vi "VoltageBlocks.vi"() -> ()   [LabVIEW 2011]
uses:
  <vilib>/DAQmx/write.llb/DAQmx Write (Analog 1D DBL NChan 1Samp).vi
  <vilib>/DAQmx/create/channels.llb/DAQmx Create Channel (AO-Voltage-Basic).vi
  <vilib>/DAQmx/miscellaneous.llb/DAQmx Fill In Error Info.vi
panel:
  in  "data":dbl[](array[slide]) scale=0.0..4.5
  in  "physical channels":tag
  out "Waveform Chart":dynamicdata(graph)
  in  "stop":bool
  in  "maximum value":dbl=5.0 format="%0.2f"
  in  "minimum value":dbl=-5.0 format="%0.2f"
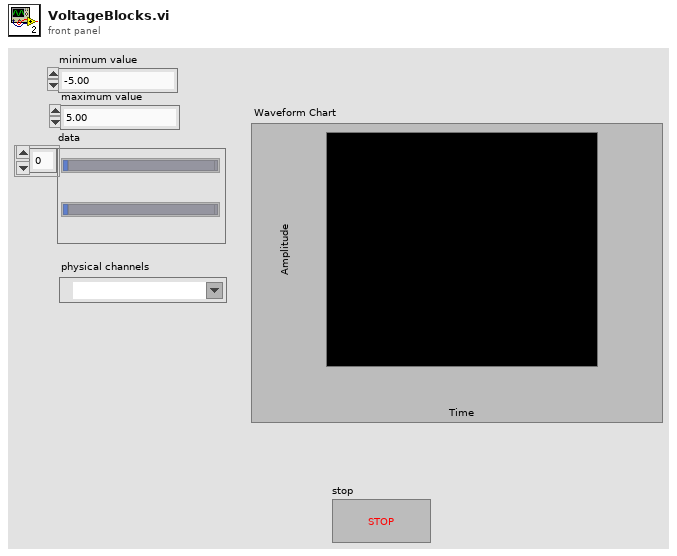
[diagram p1: front panel]
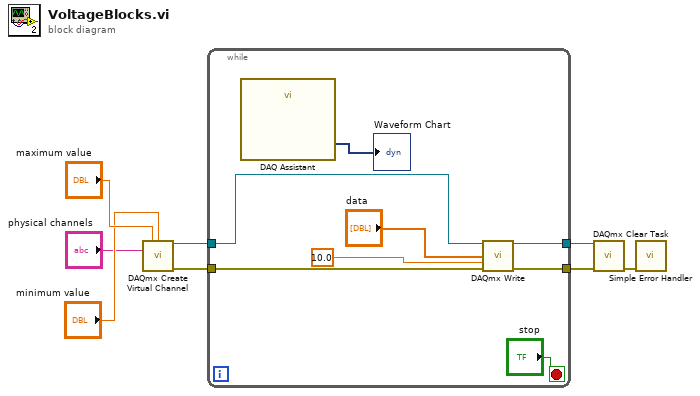
[diagram p0: block diagram]
diagram:
  n1 = call-poly <vilib>:"DAQmx Create Virtual Channel.vi"("maximum value"="maximum value", "minimum value"="minimum value", "physical channels"="physical channels") -> ("task out"=w2:refnum<k21>, "error out"=w1:errorcluster)  [unwired: 11 in]
  n2 = while {
    tunnel: [w13] -> w7
    tunnel: [w12] -> w6
    tunnel: w2 -> [w11]
    tunnel: w1 -> [w10]
    stop <- "stop" stop-if-true
    n3 = call "DAQ Assistant"() -> ("data"=→"Waveform Chart":dynamicdata)  [unwired: 17 in, 2 out]
    n4 = call-poly <vilib>:"DAQmx Write.vi"("task/channels in"=w11, "data"="data", "timeout"=10.0, "error in"=w10) -> ("task out"=w13:refnum<k21>, "error out"=w12:errorcluster)  [unwired: 9 in, 1 out]
  }
  n5 = call <vilib>:"DAQmx Clear Task.vi"("task in"=w7, "error in"=w6) -> ("error out"=w8:errorcluster)  [unwired: 13 in]
  n6 = call <vilib>:"Simple Error Handler.vi"("error in (no error)"=w8) -> ()  [unwired: 4 in, 5 out]
